vi "Sine.Generate.Convert.vi"(11 "Settings":T2) -> (3 "Settings":T1)   [LabVIEW 2019, in "Speciality FPGA IO.lvlib"]
uses:
  Speciality FPGA IO.lvlib
  Types/Sine.Generate.Convert.Settings.ctl
  Types/Sine.Generate.Settings.ctl
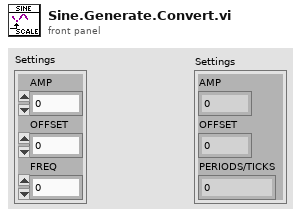
[diagram p1: front panel]
types:
  T1 = typedef "Speciality FPGA IO.lvlib/Sine.Generate.Settings.ctl" = cluster{"AMP":fxp<+/-,32,8>, "OFFSET":fxp<+/-,32,8>, "PERIODS/TICKS":fxp<+,32,0>}
  T2 = typedef "Speciality FPGA IO.lvlib/Sine.Generate.Convert.Settings.ctl" = cluster{"AMP":sgl, "OFFSET":sgl, "FREQ":sgl}
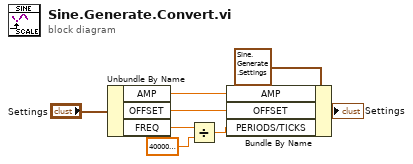
[diagram p0: block diagram]
diagram:
  n1 = Unbundle By Name("Settings") -> ("AMP"=w4:sgl, "OFFSET"=w3:sgl, "FREQ"=w2:sgl)
  n2 = Divide(x=w2, y=sgl 40000000.0) -> (x/y=w6:sgl)
  n3 = Bundle By Name(cluster=T1 {"AMP"=0.0, "OFFSET"=0.0, "PERIODS/TICKS"=0.0002500000409781933} ("Settings"), "AMP"=w4, "OFFSET"=w3, "PERIODS/TICKS"=w6) -> (→"Settings":T1)
